vi "Validate motor.vi"(6 "current code":string, 7 "enabled codes":string, 8 "error in (no error)":errorcluster, 11 "Motor in":refnum<class "Motor.lvclass">) -> (0 "error out":errorcluster, 3 "Motor out":refnum<class "Motor.lvclass">)   [LabVIEW 2018, in "Motor.lvclass"]
uses:
  Motor.lvclass
  Motor.lvclass/Motor.ctl
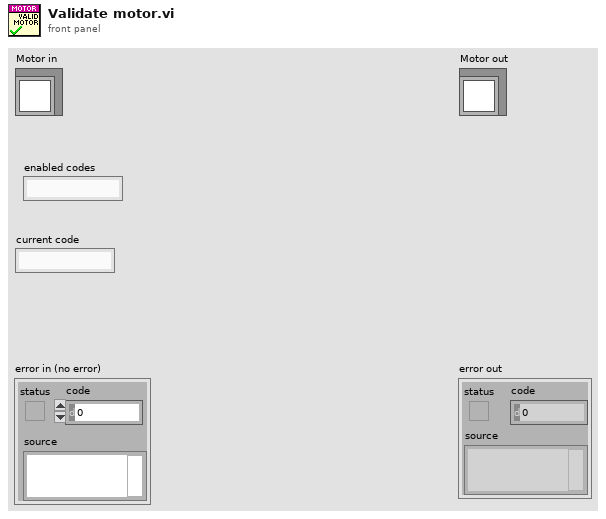
[diagram p1: front panel]
types:
  T1 = cluster{"mode":string, "condition":string, "position":string, "pos_name":string, "pos_id":string}
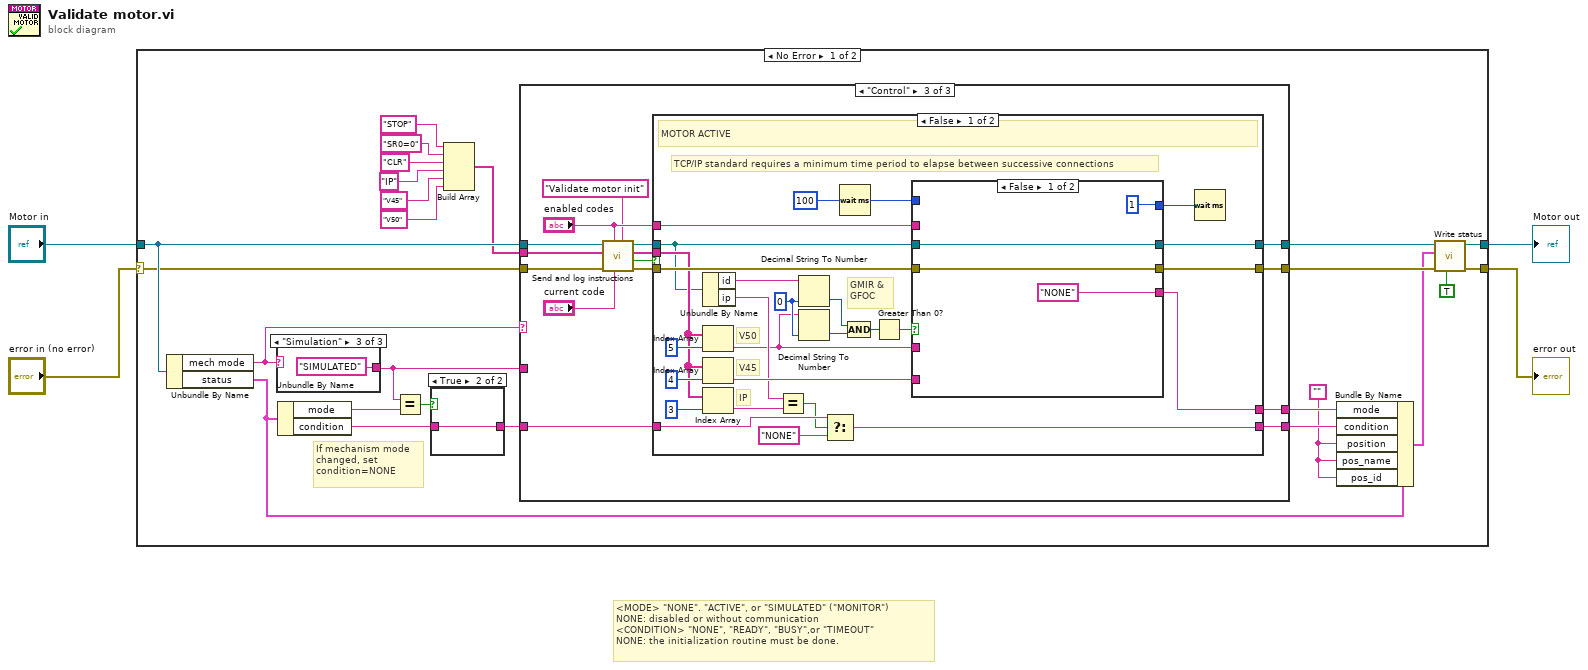
[diagram p0: block diagram]
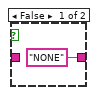
[diagram p2: hidden frame]
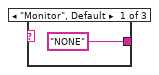
[diagram p3: hidden frame]
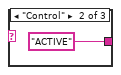
[diagram p4: hidden frame]
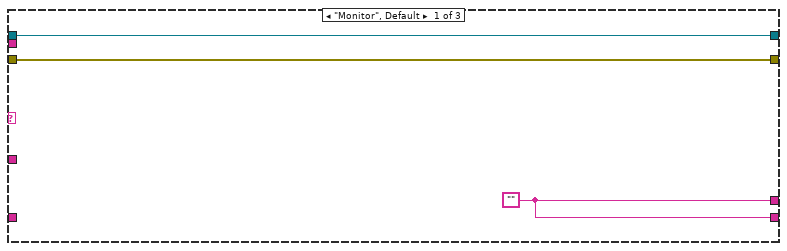
[diagram p5: hidden frame]
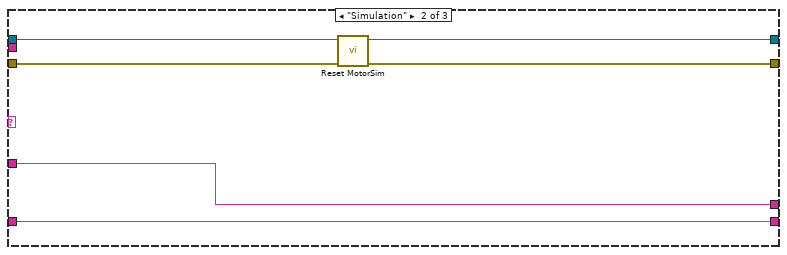
[diagram p6: hidden frame]
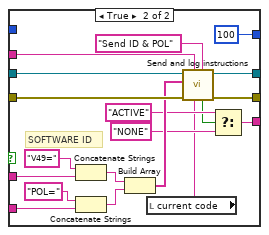
[diagram p7: hidden frame]
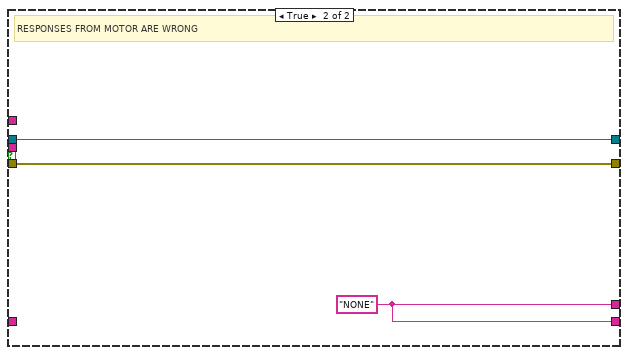
[diagram p8: hidden frame]
diagram:
  # "<MODE> \"NONE\". \"ACTIVE\", or \"SIMULATED\" (\"MONITOR\")\nNONE: disabled or without communication\n<CONDITION> \"NONE\", \"READY\", \"BUSY\",or \"TIMEOUT\"\nNONE: the initialization routine must be done."
  n1 = case shown="No Error" "error in (no error)" {
    selector: "error in (no error)" -> [w24 w112]
    tunnel: [w22 w113] -> w2
    tunnel: "Motor in" -> [w29 w113]
    tunnel: [w20 w112] -> w1
    frame No Error {
      w25 = ""
      # "If mechanism mode\nchanged, set \ncondition=NONE"
      n2 = Unbundle By Name(w29) -> ("mech mode"=w12:string, "status"=w13:T1)
      n3 = case shown="\"Simulation\"" w12 {
        tunnel: ["NONE" "ACTIVE" "SIMULATED"] -> w11
        frame "Monitor", Default {
        }
        frame "Control" {
        }
        frame "Simulation" {
        }
      }
      n4 = Unbundle By Name(w13) -> ("mode"=w16:string, "condition"=w15:string)
      n5 = Equal?(x=w11, y=w16) -> (x = y?=w17:bool)
      n6 = case shown="True" w17 {
        tunnel: ["NONE" w31] -> w14
        tunnel: w15 -> [_ w31]
        frame False {
        }
        frame True {
        }
      }
      n7 = Build Array("STOP", "SR0=0", "CLR", "IP", "V45", "V50") -> (w28:string[])
      n8 = case shown="\"Control\"" w12 {
        tunnel: w29 -> [w36 w40 w58]
        tunnel: w28 -> [_ _ w57]
        tunnel: [w37 w38 w56] -> w27
        tunnel: [w37 w43 w55] -> w26
        tunnel: [w36 w39 w54] -> w23
        tunnel: [w35 w42 w53] -> w21
        tunnel: w24 -> [w35 w41 w52]
        tunnel: w14 -> [_ w43 w51]
        tunnel: w11 -> [_ w38 _]
        frame "Monitor", Default {
          w37 = ""
        }
        frame "Simulation" {
          n9 = call-dynamic "Reset MotorSim.vi"("error in (no error)"=w41, "Motor in"=w40) -> ("error out"=w42:errorcluster, "Motor out"=w39:refnum<class "Motor.lvclass">)  [unwired: 8 in]
        }
        frame "Control" {
          n10 = call-dynamic "Send and log instructions.vi"("prefix"="Validate motor init", "current code"="current code", "enabled codes"="enabled codes", "error in (no error)"=w52, "instructions"=w57, "Motor in"=w58) -> ("error out"=w48:errorcluster, "error"=w47:bool, "replies"=w50:string[], "Motor out"=w49:refnum<class "Motor.lvclass">)  [unwired: 1 in, 1 out]
          n11 = case shown="False" w47 {
            tunnel: w50 -> [w80 _]
            tunnel: w49 -> [w74 w109]
            tunnel: w48 -> [w85 w110]
            tunnel: [w64 w111] -> w56
            tunnel: [w77 w111] -> w55
            tunnel: [w76 w109] -> w54
            tunnel: [w75 w110] -> w53
            tunnel: w51 -> [w71 _]
            tunnel: "enabled codes" -> [w62 _]
            frame False {
              w69 = u32 0 ("default (0 I32)")
              # "TCP/IP standard requires a minimum time period to elapse between successive connections"
              # "GMIR &\nGFOC"
              # "IP"
              # "V50"
              # "V45"
              # "MOTOR ACTIVE"
              n12 = Unbundle By Name(w74) -> ("id"=w70:string, "ip"=w72:string)
              n13 = Index Array(array=w80, index=5) -> (element=w68:string)
              n14 = Index Array(array=w80, index=4) -> (element=w82:string)
              n15 = Index Array(array=w80, index=3) -> (element=w73:string)
              n16 = Equal?(x=w72, y=w73) -> (x = y?=w63:bool)
              n17 = Decimal String To Number(string=w70, default (0L)=w69) -> (number=w67:u32)  [unwired: 1 in, 1 out]
              n18 = Decimal String To Number(string=w68, default (0L)=w69) -> (number=w66:u32)  [unwired: 1 in, 1 out]
              n19 = Select(t=w71, s=w63, f="NONE") -> (s? t:f=w77:string)
              n20 = Wait (ms)(milliseconds to wait=u32 100) -> (millisecond timer value=w60:u32)
              n21 = Compound Arithmetic op=AND(w67, w66) -> (w65:u32)
              n22 = Greater Than 0?(x=w65) -> (x > 0?=w79:bool)
              n23 = case shown="False" w79 {
                tunnel: w74 -> [w88 w108]
                tunnel: w85 -> [w89 w107]
                tunnel: w82 -> [_ w100]
                tunnel: [w88 w99] -> w76
                tunnel: [w89 w98] -> w75
                tunnel: w68 -> [_ w101]
                tunnel: ["NONE" w95] -> w64
                tunnel: w62 -> [_ w93]
                tunnel: w60 -> [_ _]
                tunnel: [u32 1 ("milliseconds to wait") u32 100 ("milliseconds to wait")] -> w59
                frame False {
                }
                frame True {
                  # "SOFTWARE ID"
                  n24 = Concatenate Strings("V49=", w101) -> (w104:string)
                  n25 = Concatenate Strings("POL=", w100) -> (w103:string)
                  n26 = Build Array(w104, w103) -> (w102:string[])
                  n27 = local read "current code"() -> (w91:string)
                  n28 = call-dynamic "Send and log instructions.vi"("prefix"="Send ID & POL", "current code"=w91, "enabled codes"=w93, "error in (no error)"=w107, "instructions"=w102, "Motor in"=w108) -> ("error out"=w98:errorcluster, "Motor out"=w99:refnum<class "Motor.lvclass">, "ok"=w94:bool)  [unwired: 1 in, 2 out]
                  n29 = Select(t="ACTIVE", s=w94, f="NONE") -> (s? t:f=w95:string)
                }
              }
              n30 = Wait (ms)(milliseconds to wait=w59) -> ()  [unwired: 1 out]
            }
            frame True {
              w111 = "NONE"
              # "RESPONSES FROM MOTOR ARE WRONG"
            }
          }
        }
      }
      n31 = Bundle By Name(cluster=w13, "mode"=w27, "condition"=w26, "position"=w25, "pos_name"=w25, "pos_id"=w25) -> (w19:T1)
      n32 = call-dynamic "Write status.vi"("hold if empty"=TRUE, "error in (no error)"=w21, "status"=w19, "Motor in"=w23) -> ("error out"=w20:errorcluster, "Motor out"=w22:refnum<class "Motor.lvclass">)  [unwired: 6 in]
    }
    frame Error {
    }
  }
  "error out" <- w1
  "Motor out" <- w2
